vi "Power Measurement Standard Deviation Error Code List Mode.vi"(8 "error in (no error)":errorcluster, 9 "Step Index (1)":i32=1, 10 "Instance (1)":i32=1, 11 "VISA resource name":refnum<visa-resource-name>) -> (0 "error out":errorcluster, 2 "Error Code":i32, 3 "VISA resource name out":refnum<visa-resource-name>)   [LabVIEW 2015, in "Rohde&Schwarz CMXP GPRF.lvlib"]
doc: "Returns a single-value error code for selected result.\n\nAttribute:\n-\n\nRemote-control command:\nCALCulate:GPRF:MEAS<i>:POWer:LIST:SDEViation?"
uses:
  <instrlib>/Rohde&Schwarz CMXP GPRF/Rohde&Schwarz CMXP GPRF.lvlib
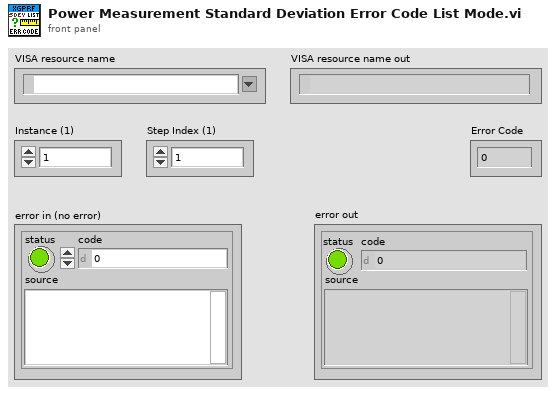
[diagram p1: front panel]
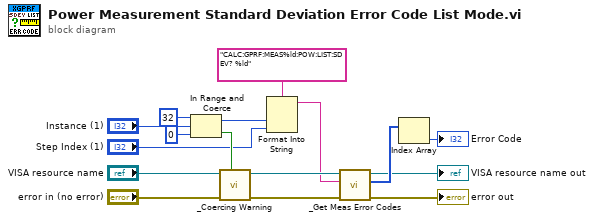
[diagram p0: block diagram]
diagram:
  n1 = In Range and Coerce(upper limit=32, x="Instance (1)", lower limit=0) -> (coerced(x)=w12:i32, In Range?=w14:bool)
  n2 = call <instrlib>:"_Coercing Warning.vi"("In Range?"=w14, "error in (no error)"="error in (no error)", "VISA resource name"="VISA resource name") -> ("error out"=w11:errorcluster, "VISA resource name out"=w10:refnum<visa-resource-name>)  [unwired: 7 in]
  n3 = Format Into String(format string="CALC:GPRF:MEAS%ld:POW:LIST:SDEV? %ld", w12, "Step Index (1)") -> (resulting string=w9:string)  [unwired: 2 in, 1 out]
  n4 = call <instrlib>:"_Get Meas Error Codes.vi"("error in (no error)"=w11, "Command"=w9, "VISA resource name"=w10) -> ("error out"=→"error out":errorcluster, "Error Codes"=w8:i32[], "VISA resource name out"=→"VISA resource name out":refnum<visa-resource-name>)  [unwired: 5 in, 1 out]
  n5 = Index Array(array=w8) -> (element=→"Error Code":i32)  [unwired: 1 in]
